vi "Get Format.vi"(8 "error in (no error)":errorcluster, 11 "Endpoint in":refnum<class "Endpoint.lvclass">) -> (0 "error out":errorcluster, 2 "Format":T1, 3 "Endpoint out":refnum<class "Endpoint.lvclass">)   [LabVIEW 2020, in "Stream-Simple-Msg.lvlib" / "Endpoint.lvclass"]
uses:
  Endpoint.lvclass
  Format.ctl
  Stream-Simple-Msg.lvlib
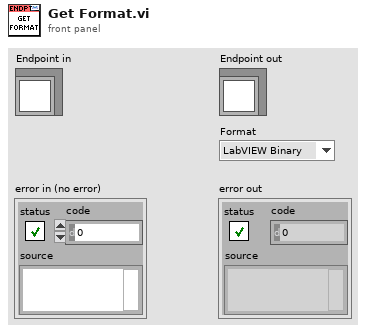
[diagram p1: front panel]
types:
  T1 = typedef "Stream-Simple-Msg.lvlib/Format.ctl" = enum16{"LabVIEW Binary", "JSON"}
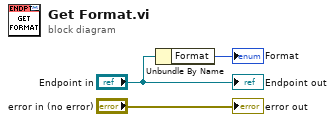
[diagram p0: block diagram]
diagram:
  n1 = Unbundle By Name("Endpoint in") -> ("Format"=→"Format":T1)
  "error out" <- "error in (no error)"
  "Endpoint out" <- "Endpoint in"
